vi "NI VeriStand - Open Single Waveform Write Session (CDB).vi"(7 "Communication Properties":T2, 8 "error in (no error)":errorcluster, 10 "dt":dbl=nan, 11 "CDB Waveform Data Reference":T1) -> (0 "error out":errorcluster, 3 "Single Waveform Write Session (CDB)":refnum<class "Single Waveform Write (CDB).lvclass">)   [LabVIEW 2020, in "NI_VS Custom Device Waveform API.lvlib" / "Single Waveform Write (CDB).lvclass"]
doc: "Opens a session for reading data from or writing data to a specific waveform or waveforms associated with a custom device. You must manually select the instance to use according to the number of waveforms with which you want to interact, whether the data type of the waveforms is DBL or CDB, and whether you want to read or write waveform data."
uses:
  Single Waveform Write (CDB).lvclass
  D:/p4/penguin/lvaddon/Veristand/master/src/LabVIEW/vilib/NI VeriStand/Custom Device Waveform API/Waveform Session.lvclass
  Communication Properties.ctl
  Custom Device API/Waveform Data Reference.ctl
  Access mode.ctl
  Internal Comm Classes/WPL Comm/WPL Comm (1D CDB)/WPL Comm (1D CDB).lvclass
  Single Waveform Write (CDB).lvclass/Single Waveform Write (CDB).ctl
  Waveform Session.lvclass/Waveform Session.ctl
  Waveform Session.lvclass
  NI_VS Custom Device Waveform API.lvlib
  Custom Device API/Custom Device API.lvlib
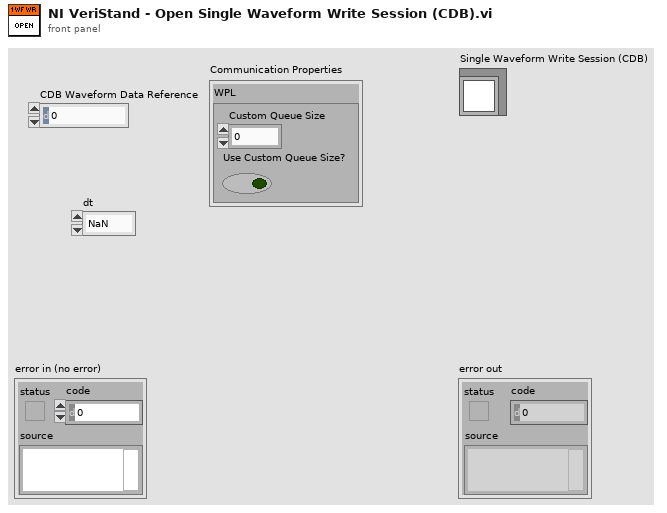
[diagram p1: front panel]
types:
  T1 = typedef "Custom Device API.lvlib/Waveform Data Reference.ctl" = i32
  T2 = typedef "NI_VS Custom Device Waveform API.lvlib/Communication Properties.ctl" = cluster{"WPL":cluster{"Custom Queue Size":i32, "Use Custom Queue Size?":bool}}
  T3 = typedef "NI_VS Custom Device Waveform API.lvlib/Access mode.ctl" = enum16{"Read", "Write"}
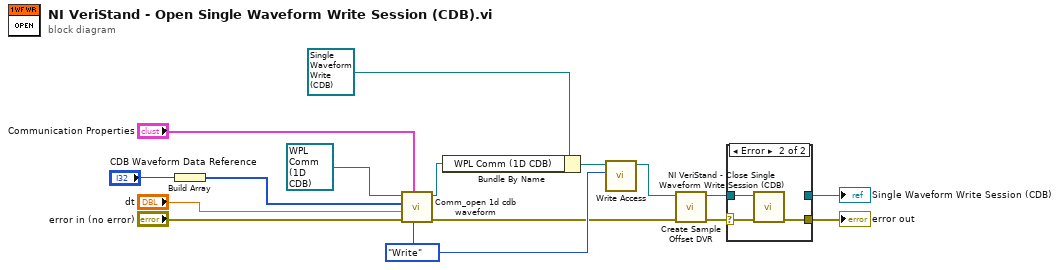
[diagram p0: block diagram]
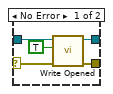
[diagram p2: hidden frame]
diagram:
  w13 = Access_mode."Write" ("Access")
  n1 = Build Array("CDB Waveform Data Reference") -> (w2:T1[])
  n2 = call "Comm_open 1d cdb waveform.vi"("Access"=w13, "Communication Properties"="Communication Properties", "error in (no error)"="error in (no error)", "dt"="dt", "Waveform Data Refs"=w2, "WPL Comm (1D CDB) in"=refnum<class "WPL Comm (1D CDB).lvclass"> refnum ("Internal Comm Classes.lvlib:WPL Comm (1D CDB).lvclass")) -> ("error out"=w12:errorcluster, "WPL Comm (1D CDB) out"=w6:refnum<class "WPL Comm (1D CDB).lvclass">)  [unwired: 4 in]
  n3 = Bundle By Name(cluster=refnum<class "Single Waveform Write (CDB).lvclass"> refnum, "WPL Comm (1D CDB)"=w6) -> (w5:refnum<class "Single Waveform Write (CDB).lvclass">)
  n4 = call "Write Access.vi"("Access"=w13, "Waveform Session in"=w5) -> ("Waveform Session out"=w9:refnum<class "Single Waveform Write (CDB).lvclass">)  [unwired: 9 in]
  n5 = call "Create Sample Offset DVR.vi"("error in (no error)"=w12, "Waveform Session in"=w9) -> ("error out"=w10:errorcluster, "Waveform Session out"=w11:refnum<class "Single Waveform Write (CDB).lvclass">)  [unwired: 8 in]
  n6 = case shown="Error" w10 {
    selector: w10 -> [w20 w23]
    tunnel: [w20 w22] -> w16
    tunnel: w11 -> [w19 w21]
    tunnel: [w18 _] -> w14
    frame No Error {
      n7 = call "Write Opened.vi"("Opened"=TRUE, "Waveform Session in"=w19) -> ("Waveform Session out"=w18:refnum<class "Single Waveform Write (CDB).lvclass">)  [unwired: 9 in]
    }
    frame Error {
      n8 = call "NI VeriStand - Close Single Waveform Write Session (CDB).vi"("error in (no error)"=w23, "Single Waveform Write Session (CDB)"=w21) -> ("error out"=w22:errorcluster)  [unwired: 9 in]
    }
  }
  "error out" <- w16
  "Single Waveform Write Session (CDB)" <- w14
